vi "DEMO.vi"() -> ()   [LabVIEW 2013]
panel:
  out "Lamp":bool[](array[boolean])
  in  "停止":bool
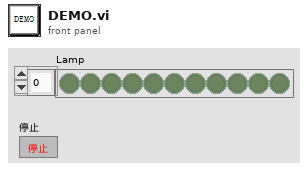
[diagram p1: front panel]
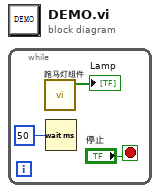
[diagram p0: block diagram]
diagram:
  n1 = while {
    stop <- "停止" stop-if-true
    n2 = call "跑马灯组件.vi"() -> ("Lamp"=→"Lamp":bool[])  [unwired: 9 in, 1 out]
    n3 = Wait (ms)(milliseconds to wait=u32 50 ("等待时间（毫秒）")) -> ()  [unwired: 1 out]
  }
